vi "Write 1Port 1Samp 1D Boolean.vi"(8 "error in (no error)":errorcluster, 9 "value":u8 format="%08b", 10 "Port (Bank)":T1 items=["DIO1...8"=1, "DIO9...16"=2, "DIO17...24"=3, "DIO25...32"=4], 11 "MicroDAQ.lvlib:Digital output.lvclass":refnum<class "Digital output.lvclass">) -> (0 "error out":errorcluster, 3 "MicroDAQ.lvlib:Digital output.lvclass out":refnum<class "Digital output.lvclass">)   [LabVIEW 2009, in "MicroDAQ.lvlib" / "Digital output.lvclass"]
doc: "Writes a single U8 register value to a digital output channel composed of a single port."
uses:
  <instrlib>/MicroDAQ/Channel/Digital output/Digital output.lvclass
  <instrlib>/MicroDAQ/Tools/Digital IO channels.ctl
  <instrlib>/MicroDAQ/MicroDAQ.lvlib
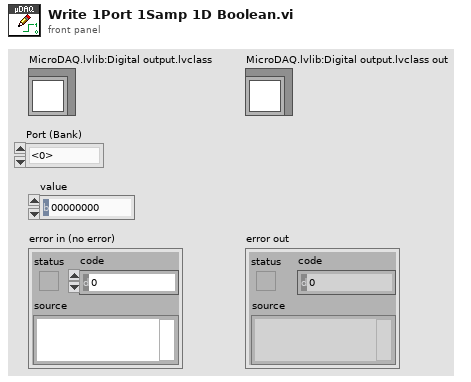
[diagram p1: front panel]
types:
  T1 = typedef "MicroDAQ.lvlib/Digital IO channels.ctl" = u8
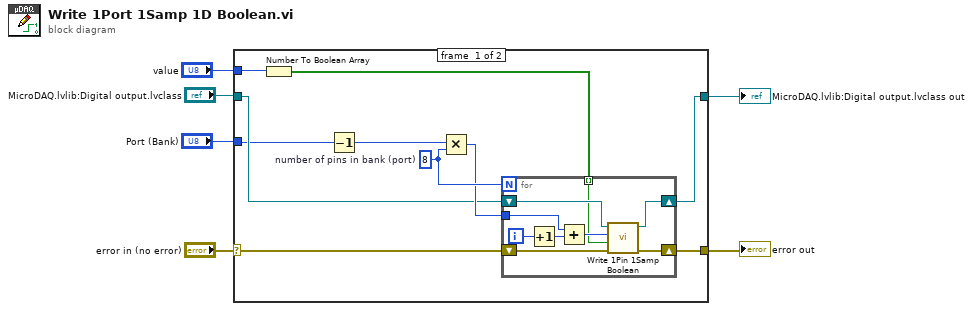
[diagram p0: block diagram]
diagram:
  n1 = case shown="No Error" "error in (no error)" {
    selector: "error in (no error)" -> [w14 w26]
    tunnel: [w13 w26] -> w5
    tunnel: "MicroDAQ.lvlib:Digital output.lvclass" -> [w12 w27]
    tunnel: [w11 w27] -> w3
    tunnel: "Port (Bank)" -> [w10 _]
    tunnel: "value" -> [w9 _]
    frame #0 {
      w16 = 8  # number of pins in bank (port)
      n2 = Number To Boolean Array(number=w9) -> (Boolean array=w7:bool[])
      n3 = Decrement(x=w10) -> (x-1=w8:T1)
      n4 = Multiply(x=w8, y=w16) -> (x*y=w15:i32)
      n5 = for {
        N: w16 -> [_]
        shift-right: [w19] -> w13
        shift-left: w14 -> [w23]
        tunnel: w15 -> [w24]
        shift-right: [w20] -> w11
        shift-left: w12 -> [w21]
        tunnel: w7 -> [w18] mode=indexing
        i -> [w25]
        n6 = Increment(x=w25) -> (x+1=w17:i32)
        n7 = Add(x=w24, y=w17) -> (x+y=w22:i32)
        n8 = call <instrlib>:"Write 1Pin 1Samp Boolean.vi"("error in (no error)"=w23, "data"=w18, "Pin"=w22, "MicroDAQ.lvlib:Digital output.lvclass"=w21) -> ("error out"=w19:errorcluster, "MicroDAQ.lvlib:Digital output.lvclass out"=w20:refnum<class "Digital output.lvclass">)  [unwired: 6 in]
      }
    }
    frame #1 {
    }
  }
  "error out" <- w5
  "MicroDAQ.lvlib:Digital output.lvclass out" <- w3
